vi "ble_cmd_attclient_attribute_write.vi"(4 "data (uint8array)":u8[](array[numeric]) format="%02x", 6 "Connection Status":T1={"MAC Address"="", "cnx handle"=0, "cnx flags"=0, "Address Type"=125, "Connection Interval (ms)"=125, "Timeout(ms)"=125, "Latency"=0, "bonding handle"=0} {"Address Type" items=["Public", "Random"]}, 7 "chrHandle":u16=1 format="%04x", 8 "error in (no error)":errorcluster, 11 "COM Bluegiga in":refnum<visa-resource-name>) -> (0 "error out":errorcluster, 3 "COM Bluegiga out":refnum<visa-resource-name>)   [LabVIEW 2015]
uses:
  type_def/connection_status_bundle.ctl
  type_def/address_type.ctl
  type_def/message_class.ctl
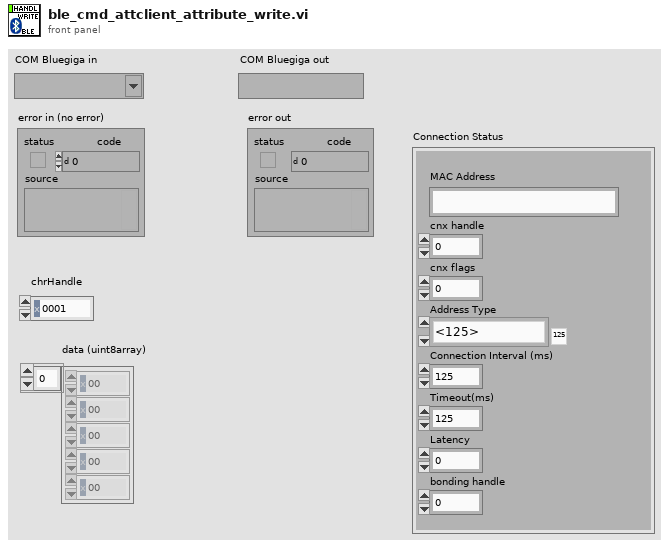
[diagram p1: front panel]
types:
  T1 = typedef "connection_status_bundle.ctl" = cluster{"MAC Address":string, "cnx handle":u8, "cnx flags":u8, "Address Type":T2, "Connection Interval (ms)":u16, "Timeout(ms)":u16, "Latency":u16, "bonding handle":u8}
  T2 = typedef "address_type.ctl" = u8
  T3 = typedef "message_class.ctl" = u8
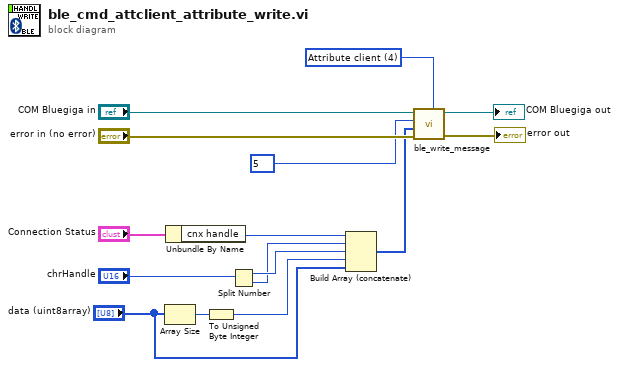
[diagram p0: block diagram]
diagram:
  w6 = T3 4 items=["System", "Persistent Store", "Attribute database", "Connection", "Attribute client", "Security Manager", "Generic Access Profile", "Hardware"] ("Command Class (System)")
  n1 = Array Size(array="data (uint8array)") -> (size(s)=w3:i32)
  n2 = Unbundle By Name("Connection Status") -> ("cnx handle"=w11:u8)
  n3 = To Unsigned Byte Integer(number=w3) -> (unsigned 8bit integer=w2:u8)
  n4 = Split Number(x="chrHandle") -> (hi(x)=w8:u8, lo(x)=w7:u8)
  n5 = Build Array (concatenate)(w11, w7, w8, w2, "data (uint8array)") -> (w10:u8[])
  n6 = call "ble_write_message.vi"("Command Class (System)"=w6, "error in (no error)"="error in (no error)", "Payload(Empty)"=w10, "Message ID (0x00)"=u8 5, "COM Bluegiga in"="COM Bluegiga in") -> ("error out"=→"error out":errorcluster, "COM Bluegiga out"=→"COM Bluegiga out":refnum<visa-resource-name>)  [unwired: 4 in, 1 out]
